vi "Monitor Switches.vi"(8 "error in (no error)":errorcluster, 10 "Switches":bool[](array[boolean]), 11 "Attributes in":refnum<class "Attributes.lvclass">) -> (0 "error out":errorcluster, 2 "Indicators":T1, 3 "Attributes out":refnum<class "Attributes.lvclass">)   [LabVIEW 2021, in "Attributes.lvclass"]
uses:
  Attributes.lvclass
  Attributes.lvclass/Attributes.ctl
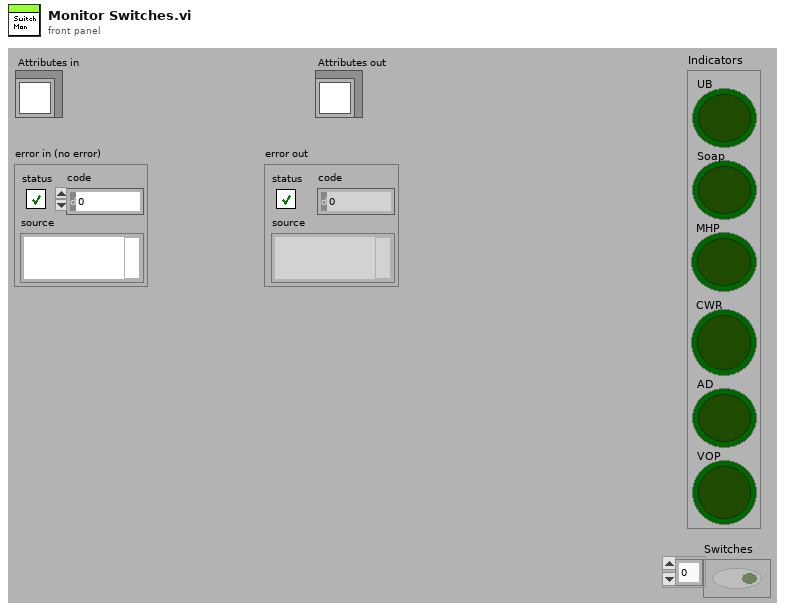
[diagram p1: front panel]
types:
  T1 = cluster{"UB":bool, "Soap":bool, "MHP":bool, "CWR":bool, "AD":bool, "VOP":bool}
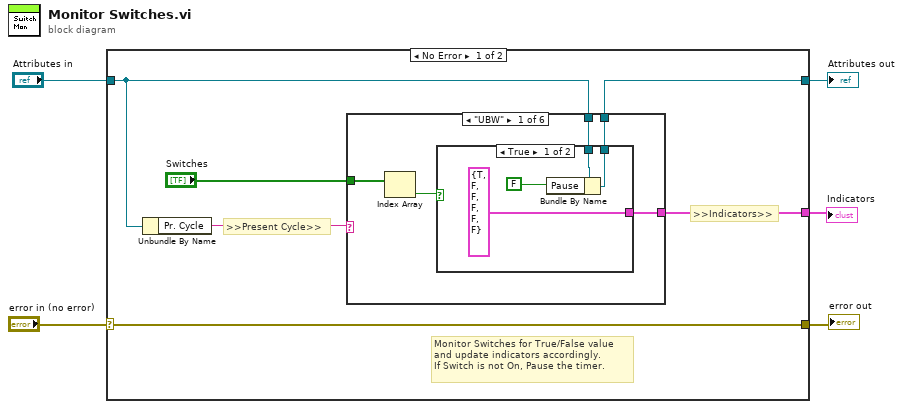
[diagram p0: block diagram]
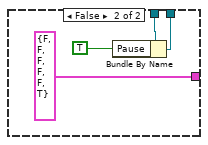
[diagram p2: hidden frame]
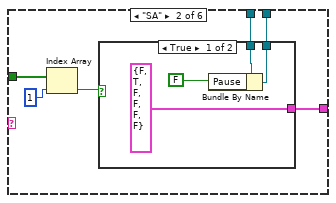
[diagram p3: hidden frame]
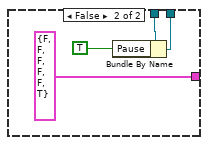
[diagram p4: hidden frame]
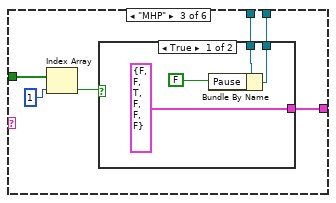
[diagram p5: hidden frame]
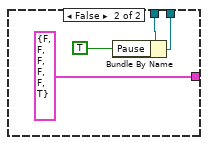
[diagram p6: hidden frame]
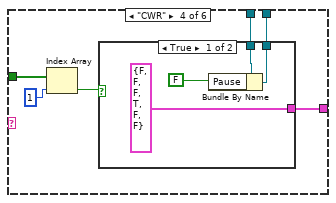
[diagram p7: hidden frame]
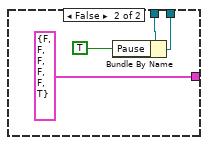
[diagram p8: hidden frame]
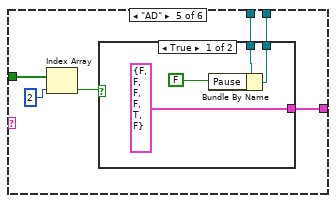
[diagram p9: hidden frame]
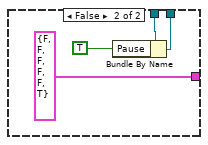
[diagram p10: hidden frame]
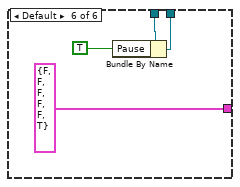
[diagram p11: hidden frame]
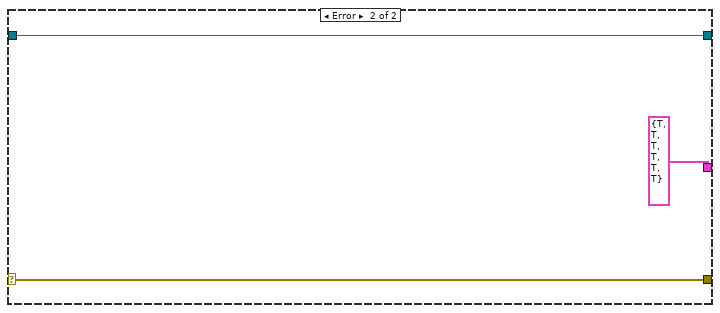
[diagram p12: hidden frame]
diagram:
  n1 = case shown="No Error" "error in (no error)" {
    selector: "error in (no error)" -> [w11 w87]
    tunnel: [w11 w87] -> w4
    tunnel: [w6 w86] -> w2
    tunnel: "Attributes in" -> [w7 w86]
    tunnel: [w8 T1 {"UB"=TRUE, "Soap"=TRUE, "MHP"=TRUE, "CWR"=TRUE, "AD"=TRUE, "VOP"=TRUE} ("Ind.")] -> w1
    frame No Error {
      # "Monitor Switches for True/False value\nand update indicators accordingly.\nIf Switch is not On, Pause the timer."
      # ">>Indicators>>"
      # ">>Present Cycle>>"
      n2 = Unbundle By Name(w7) -> ("Pr. Cycle"=w10:string)
      n3 = case shown="\"UBW\"" w10 {
        tunnel: [w16 w30 w44 w58 w72 T1 {"UB"=FALSE, "Soap"=FALSE, "MHP"=FALSE, "CWR"=FALSE, "AD"=FALSE, "VOP"=TRUE} ("Ind.")] -> w8
        tunnel: "Switches" -> [w15 w29 w43 w57 w71 _]
        tunnel: w7 -> [w13 w27 w41 w55 w69 w83]
        tunnel: [w12 w26 w40 w54 w68 w82] -> w6
        frame "UBW" {
          n4 = Index Array(array=w15) -> (element=w14:bool)  [unwired: 1 in]
          n5 = case shown="True" w14 {
            tunnel: [T1 {"UB"=TRUE, "Soap"=FALSE, "MHP"=FALSE, "CWR"=FALSE, "AD"=FALSE, "VOP"=FALSE} ("Ind.") T1 {"UB"=FALSE, "Soap"=FALSE, "MHP"=FALSE, "CWR"=FALSE, "AD"=FALSE, "VOP"=TRUE} ("Ind.")] -> w16
            tunnel: w13 -> [w19 w23]
            tunnel: [w18 w22] -> w12
            frame True {
              n6 = Bundle By Name(cluster=w19, "Pause"=FALSE) -> (w18:refnum<class "Attributes.lvclass">)
            }
            frame False {
              n7 = Bundle By Name(cluster=w23, "Pause"=TRUE) -> (w22:refnum<class "Attributes.lvclass">)
            }
          }
        }
        frame "SA" {
          n8 = Index Array(array=w29, index=1) -> (element=w28:bool)
          n9 = case shown="True" w28 {
            tunnel: [T1 {"UB"=FALSE, "Soap"=TRUE, "MHP"=FALSE, "CWR"=FALSE, "AD"=FALSE, "VOP"=FALSE} ("Ind.") T1 {"UB"=FALSE, "Soap"=FALSE, "MHP"=FALSE, "CWR"=FALSE, "AD"=FALSE, "VOP"=TRUE} ("Ind.")] -> w30
            tunnel: w27 -> [w33 w37]
            tunnel: [w32 w36] -> w26
            frame True {
              n10 = Bundle By Name(cluster=w33, "Pause"=FALSE) -> (w32:refnum<class "Attributes.lvclass">)
            }
            frame False {
              n11 = Bundle By Name(cluster=w37, "Pause"=TRUE) -> (w36:refnum<class "Attributes.lvclass">)
            }
          }
        }
        frame "MHP" {
          n12 = Index Array(array=w43, index=1) -> (element=w42:bool)
          n13 = case shown="True" w42 {
            tunnel: [T1 {"UB"=FALSE, "Soap"=FALSE, "MHP"=TRUE, "CWR"=FALSE, "AD"=FALSE, "VOP"=FALSE} ("Ind.") T1 {"UB"=FALSE, "Soap"=FALSE, "MHP"=FALSE, "CWR"=FALSE, "AD"=FALSE, "VOP"=TRUE} ("Ind.")] -> w44
            tunnel: w41 -> [w47 w51]
            tunnel: [w46 w50] -> w40
            frame True {
              n14 = Bundle By Name(cluster=w47, "Pause"=FALSE) -> (w46:refnum<class "Attributes.lvclass">)
            }
            frame False {
              n15 = Bundle By Name(cluster=w51, "Pause"=TRUE) -> (w50:refnum<class "Attributes.lvclass">)
            }
          }
        }
        frame "CWR" {
          n16 = Index Array(array=w57, index=1) -> (element=w56:bool)
          n17 = case shown="True" w56 {
            tunnel: [T1 {"UB"=FALSE, "Soap"=FALSE, "MHP"=FALSE, "CWR"=TRUE, "AD"=FALSE, "VOP"=FALSE} ("Ind.") T1 {"UB"=FALSE, "Soap"=FALSE, "MHP"=FALSE, "CWR"=FALSE, "AD"=FALSE, "VOP"=TRUE} ("Ind.")] -> w58
            tunnel: w55 -> [w61 w65]
            tunnel: [w60 w64] -> w54
            frame True {
              n18 = Bundle By Name(cluster=w61, "Pause"=FALSE) -> (w60:refnum<class "Attributes.lvclass">)
            }
            frame False {
              n19 = Bundle By Name(cluster=w65, "Pause"=TRUE) -> (w64:refnum<class "Attributes.lvclass">)
            }
          }
        }
        frame "AD" {
          n20 = Index Array(array=w71, index=2) -> (element=w70:bool)
          n21 = case shown="True" w70 {
            tunnel: [T1 {"UB"=FALSE, "Soap"=FALSE, "MHP"=FALSE, "CWR"=FALSE, "AD"=TRUE, "VOP"=FALSE} ("Ind.") T1 {"UB"=FALSE, "Soap"=FALSE, "MHP"=FALSE, "CWR"=FALSE, "AD"=FALSE, "VOP"=TRUE} ("Ind.")] -> w72
            tunnel: w69 -> [w75 w79]
            tunnel: [w74 w78] -> w68
            frame True {
              n22 = Bundle By Name(cluster=w75, "Pause"=FALSE) -> (w74:refnum<class "Attributes.lvclass">)
            }
            frame False {
              n23 = Bundle By Name(cluster=w79, "Pause"=TRUE) -> (w78:refnum<class "Attributes.lvclass">)
            }
          }
        }
        frame Default {
          n24 = Bundle By Name(cluster=w83, "Pause"=TRUE) -> (w82:refnum<class "Attributes.lvclass">)
        }
      }
    }
    frame Error {
    }
  }
  "error out" <- w4
  "Attributes out" <- w2
  "Indicators" <- w1
